vi "Replace Outside Typedef Const.vi"(6 "dependent vis":path[](array[path]), 8 "error in":errorcluster, 9 "shared directory":path, 10 "non-library vi[]":string[](array[string]), 11 "measurement directory":path) -> (0 "error out":errorcluster)   [LabVIEW 2021, in "Multiple Converter.lvlib"]
uses:
  Multiple Converter.lvlib
  <vilib>/Utility/traverseref.llb/TRef TravTarget.ctl
  <vilib>/Utility/traverseref.llb/VI Scripting - Traverse.lvlib
  Converter Reusables/Converter Reusables.lvlib
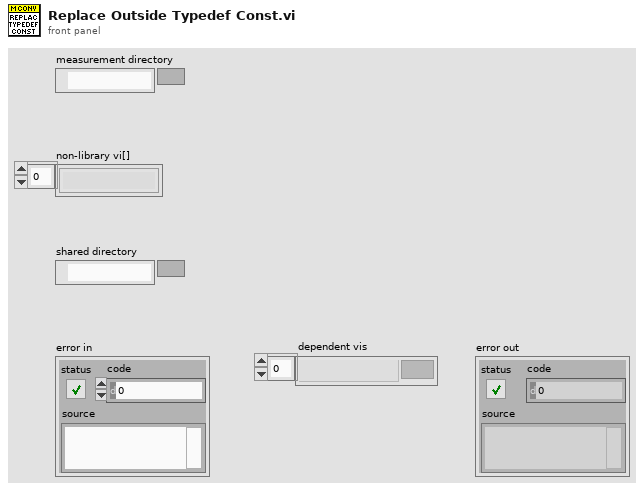
[diagram p1: front panel]
types:
  T1 = typedef "TRef TravTarget.ctl" = enum16{"FP", "BD", "Other"}
  T2 = enum32{"not a typedef", "typedef", "strict typedef", "class private data"}
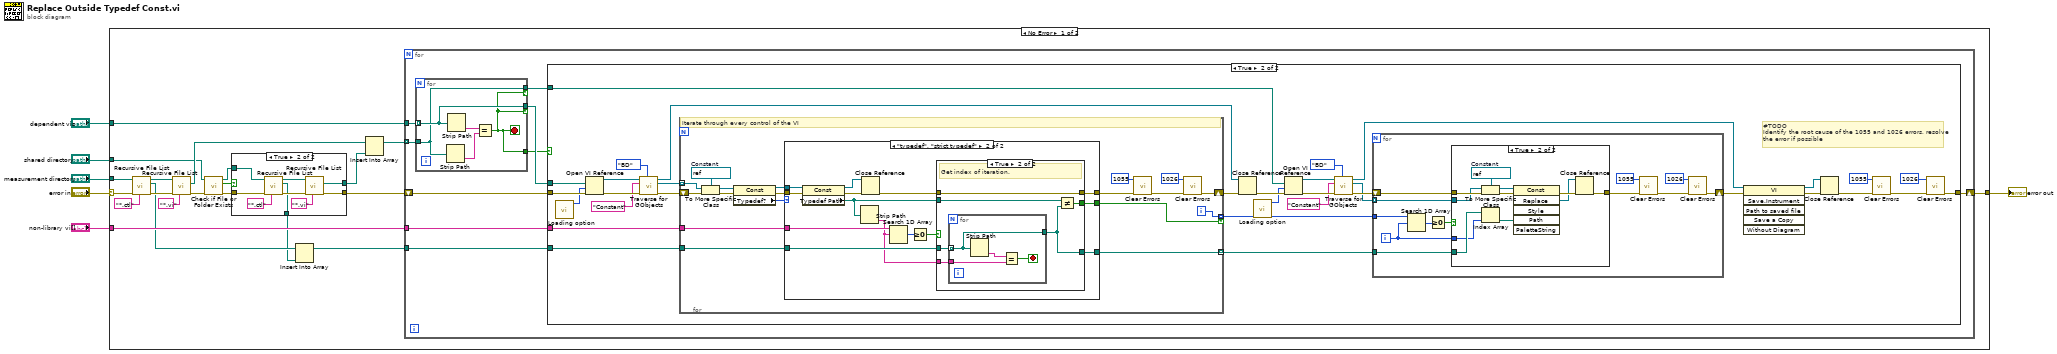
[diagram p0: block diagram]
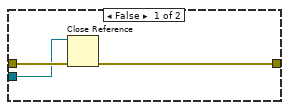
[diagram p3: hidden frame]
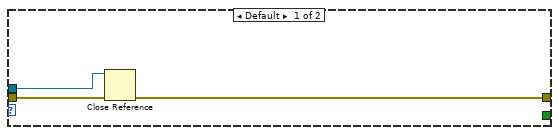
[diagram p4: hidden frame]
diagram:
  n1 = case shown="No Error" "error in" {
    selector: "error in" -> [w26 w158]
    tunnel: "non-library vi[]" -> [w27 _]
    tunnel: [w24 w158] -> w4
    tunnel: "measurement directory" -> [w22 _]
    tunnel: "shared directory" -> [w8 _]
    tunnel: "dependent vis" -> [w7 _]
    frame No Error {
      n2 = call <vilib>:"Recursive File List.vi"("pattern"="*.ctl", "error in (no error)"=w26, "Folder Path"=w22) -> ("error out"=w23:errorcluster, "All Files in Dir"=w19:path[], "dup Folder Path"=w21:path)  [unwired: 4 in, 2 out]
      n3 = call <vilib>:"Recursive File List.vi"("pattern"="*.vi", "error in (no error)"=w23, "Folder Path"=w21) -> ("error out"=w17:errorcluster, "All Files in Dir"=w16:path[])  [unwired: 4 in, 3 out]
      n4 = call <vilib>:"Check if File or Folder Exists.vi"("error in (no error)"=w17, "path"=w8) -> ("error out"=w11:errorcluster, "file or folder exists?"=w10:bool, "dup path"=w9:path)  [unwired: 7 in]
      n5 = case shown="True" w10 {
        tunnel: [w148 w153] -> w18
        tunnel: w11 -> [w148 w152]
        tunnel: [_ w151] -> w13
        tunnel: [_ w150] -> w12
        tunnel: w9 -> [_ w149]
        frame False {
        }
        frame True {
          n6 = call <vilib>:"Recursive File List.vi"("pattern"="*.ctl", "error in (no error)"=w152, "Folder Path"=w149) -> ("error out"=w155:errorcluster, "All Files in Dir"=w151:path[], "dup Folder Path"=w156:path)  [unwired: 4 in, 2 out]
          n7 = call <vilib>:"Recursive File List.vi"("pattern"="*.vi", "error in (no error)"=w155, "Folder Path"=w156) -> ("error out"=w153:errorcluster, "All Files in Dir"=w150:path[])  [unwired: 4 in, 3 out]
        }
      }
      n8 = Insert Into Array(array=w19, new element=w13) -> (w14:path[])  [unwired: 1 in]
      n9 = Insert Into Array(array=w16, new element=w12) -> (w15:path[])  [unwired: 1 in]
      n10 = for {
        tunnel: w14 -> [w36]
        tunnel: w27 -> [w35]
        tunnel: w15 -> [w33] mode=indexing
        shift-right: [w29] -> w24
        shift-left: w18 -> [w31]
        tunnel: w7 -> [w34]
        n11 = for {
          tunnel: w34 -> [w145] mode=indexing
          tunnel: w33 -> [w144]
          tunnel: [w145] -> w32 if=w143
          tunnel: [w144] -> w30 if=w143
          tunnel: [w143] -> w28
          stop <- w143 stop-if-true
          n12 = Strip Path(path=w144) -> (name=w146:string)  [unwired: 1 out]
          n13 = Strip Path(path=w145) -> (name=w147:string)  [unwired: 1 out]
          n14 = Equal?(x=w147, y=w146) -> (x = y?=w143:bool)
        }
        n15 = case shown="True" w28 {
          tunnel: w36 -> [_ w70]
          tunnel: w35 -> [_ w69]
          tunnel: w32 -> [_ w65]
          tunnel: w31 -> [w37 w64]
          tunnel: w30 -> [_ w54]
          tunnel: [w37 w60] -> w29
          frame False {
          }
          frame True {
            # "#TODO\nIdentify the root cause of the 1055 and 1026 errors, resolve \nthe error if possible"
            n16 = call "Loading option.vi"() -> ("options"=w39:i32)  [unwired: 11 in]
            n17 = Open VI Reference(vi path=w65, options=w39, error in (no error)=w64) -> (vi reference=w50:refnum<vi>, error out=w62:errorcluster)  [unwired: 3 in]
            n18 = call <vilib>:"Traverse for GObjects.vi"("Traverse Target"=TRef_TravTarget."BD", "error in (no error)"=w62, "Class Name"="Constant", "VI Refnum"=w50) -> ("error out"=w51:errorcluster, "References"=w47:refnum<vi>[], "dup VI Refnum"=w46:refnum<vi>)  [unwired: 4 in, 1 out]
            n19 = for {
              tunnel: w69 -> [w112]
              tunnel: w70 -> [w114]
              shift-right: [w102] -> w56
              shift-left: w51 -> [w107]
              tunnel: [w100] -> w52 mode=indexing
              tunnel: [w98] -> w53 mode=indexing if=w99
              tunnel: w47 -> [w97] mode=indexing
              i -> [w98]
              w113 = refnum<vi> refnum  # Constant
              # "Iterate through every control of the VI"
              n20 = To More Specific Class(target class=w113, reference=w97, error in=w107) -> (specific class reference=w111:refnum<vi>, error out=w101:errorcluster)
              n21 = property class="Const"(reference=w111, error in=w101) -> (reference out=w109:refnum<vi>, error out=w110:errorcluster, "Typedef?"=w108:T2)
              n22 = case shown="\"typedef\", \"strict typedef\"" w108 {
                tunnel: w110 -> [w117 w121]
                tunnel: w109 -> [w115 w126]
                tunnel: [w116 w130] -> w106
                tunnel: w114 -> [_ w128]
                tunnel: w112 -> [_ w127]
                tunnel: [_ w119] -> w100
                tunnel: [_ w118] -> w99
                frame Default {
                  n23 = Close Reference(reference=w115, error in (no error)=w117) -> (error out=w116:errorcluster)
                }
                frame "typedef", "strict typedef" {
                  n24 = property class="Const"(reference=w126, error in=w121) -> (reference out=w122:refnum<vi>, error out=w123:errorcluster, "Typedef Path"=w124:path)
                  n25 = Strip Path(path=w124) -> (name=w125:string)  [unwired: 1 out]
                  n26 = Close Reference(reference=w122, error in (no error)=w123) -> (error out=w120:errorcluster)
                  n27 = Search 1D Array(1D array=w127, element=w125) -> (index of element=w131:i32)  [unwired: 1 in]
                  n28 = Greater Or Equal To 0?(x=w131) -> (x >= 0?=w129:bool)
                  n29 = case shown="True" w129 {
                    tunnel: [w132 w136] -> w130
                    tunnel: w128 -> [_ w138]
                    tunnel: w125 -> [_ w137]
                    tunnel: w124 -> [_ w135]
                    tunnel: w120 -> [w132 w136]
                    tunnel: [_ w134] -> w119
                    tunnel: [_ w133] -> w118
                    frame False {
                      # "Pass"
                    }
                    frame True {
                      # "Get index of iteration."
                      n30 = for {
                        tunnel: w138 -> [w139] mode=indexing
                        tunnel: w137 -> [w141]
                        tunnel: [w139] -> w134
                        stop <- w140 stop-if-true
                        n31 = Strip Path(path=w139) -> (name=w142:string)  [unwired: 1 out]
                        n32 = Equal?(x=w142, y=w141) -> (x = y?=w140:bool)
                      }
                      n33 = Not Equal?(x=w135, y=w134) -> (x != y?=w133:bool)
                    }
                  }
                }
              }
              n34 = call <vilib>:"Clear Errors.vi"("error in (no error)"=w106, "specific error code to clear (0: all)"=1055) -> ("error out"=w105:errorcluster)  [unwired: 4 in, 1 out]
              n35 = call <vilib>:"Clear Errors.vi"("error in (no error)"=w105, "specific error code to clear (0: all)"=1026) -> ("error out"=w102:errorcluster)  [unwired: 4 in, 1 out]
            }
            n36 = Close Reference(reference=w46, error in (no error)=w56) -> (error out=w63:errorcluster)
            n37 = call "Loading option.vi"() -> ("options"=w38:i32)  [unwired: 11 in]
            n38 = Open VI Reference(vi path=w54, options=w38, error in (no error)=w63) -> (vi reference=w44:refnum<vi>, error out=w55:errorcluster)  [unwired: 3 in]
            n39 = call <vilib>:"Traverse for GObjects.vi"("Traverse Target"=TRef_TravTarget."BD", "error in (no error)"=w55, "Class Name"="Constant", "VI Refnum"=w44) -> ("error out"=w45:errorcluster, "References"=w42:refnum<vi>[], "dup VI Refnum"=w43:refnum<vi>)  [unwired: 4 in, 1 out]
            n40 = for {
              tunnel: w42 -> [w78] mode=indexing
              shift-right: [w74] -> w61
              shift-left: w45 -> [w82]
              tunnel: w53 -> [w80]
              tunnel: w52 -> [w76]
              i -> [w71]
              n41 = Search 1D Array(1D array=w80, element=w71) -> (index of element=w77:i32)  [unwired: 1 in]
              n42 = Greater Or Equal To 0?(x=w77) -> (x >= 0?=w79:bool)
              n43 = case shown="True" w79 {
                tunnel: w82 -> [w85 w96]
                tunnel: [w84 w92] -> w81
                tunnel: w78 -> [w83 w90]
                tunnel: w76 -> [_ w89]
                tunnel: w71 -> [_ w86]
                frame False {
                  n44 = Close Reference(reference=w83, error in (no error)=w85) -> (error out=w84:errorcluster)
                }
                frame True {
                  w87 = refnum<vi> refnum  # Constant
                  n45 = To More Specific Class(target class=w87, reference=w90, error in=w96) -> (specific class reference=w93:refnum<vi>, error out=w95:errorcluster)
                  n46 = Index Array(array=w89, index=w86) -> (element=w88:path)
                  n47 = invoke class="Const" method="Replace"(reference=w93, error in=w95, "Path"=w88) -> (error out=w94:errorcluster, "Replace"=w91:refnum<vi>)  [unwired: 3 in, 4 out]
                  n48 = Close Reference(reference=w91, error in (no error)=w94) -> (error out=w92:errorcluster)
                }
              }
              n49 = call <vilib>:"Clear Errors.vi"("error in (no error)"=w81, "specific error code to clear (0: all)"=1055) -> ("error out"=w75:errorcluster)  [unwired: 4 in, 1 out]
              n50 = call <vilib>:"Clear Errors.vi"("error in (no error)"=w75, "specific error code to clear (0: all)"=1026) -> ("error out"=w74:errorcluster)  [unwired: 4 in, 1 out]
            }
            n51 = invoke class="VI" method="Save.Instrument"(reference=w43, error in=w61) -> (reference out=w66:refnum<vi>, error out=w67:errorcluster)  [unwired: 4 in, 4 out]
            n52 = Close Reference(reference=w66, error in (no error)=w67) -> (error out=w68:errorcluster)
            n53 = call <vilib>:"Clear Errors.vi"("error in (no error)"=w68, "specific error code to clear (0: all)"=1055) -> ("error out"=w58:errorcluster)  [unwired: 4 in, 1 out]
            n54 = call <vilib>:"Clear Errors.vi"("error in (no error)"=w58, "specific error code to clear (0: all)"=1026) -> ("error out"=w60:errorcluster)  [unwired: 4 in, 1 out]
          }
        }
      }
    }
    frame Error {
    }
  }
  "error out" <- w4
